vi "UV-VIS GetStatus.vi"(4 "error in (no error)":errorcluster, 7 "Detector in":refnum<class "CCD_camera.lvclass">) -> (0 "error out":errorcluster, 1 "DLL error code":u32, 2 "status":T1, 3 "Detector out":refnum<class "CCD_camera.lvclass">)   [LabVIEW 2018, in "CCD_camera.lvclass"]
doc: "This function will return the current status of the drivers. This function should be called before an acquisition is started to ensure that it is IDLE and during an acquisition to monitor the process.\n\n<B>Parameter:</B>\nstatus - current status\n DRV_IDLE - IDLE waiting on instructions.\n DRV_TEMPCYCLE - Executing temperature cycle.\n DRV_ACQUIRING - Acquisition in progress.\n DRV_ACCUM_TIME_NOT_MET - Unable to meet Accumulate cycle time.\n DRV_KINETIC_TIME_NOT_MET - Unable to meet Kinetic cycle time.\n DRV_ERROR_ACK - Unable to communicate with card.\n DRV_ACQ_BUFFER - Computer unable to read the data via the ISA slot at the required rate.\n\n<B>Error codes:</B>\nDRV_SUCCESS - Driver status return\nDRV_NOT_INITIALIZED - System not initialized\n\n<B>NOTES:</B>\n<B>If the status is DRV_ACCUM_TIME_NOT_MET, DRV_KINETIC_TIME_NOT_MET, DRV_ERROR_ACK or DRV_ACQ_BUFFER then the current acquisition will be aborted automatically.</B>"
uses:
  CCD_camera.lvclass
  dependecies/Error Code Enum typedef.ctl
  C:/Users/Sergey Denisov/Documents/REPS/TRANCON/Classes/Detector/Detector.lvclass
  Detector.lvclass/Detector.ctl
  Detector.lvclass
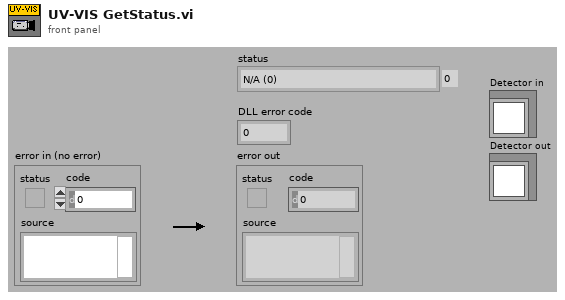
[diagram p1: front panel]
types:
  T1 = typedef "Error Code Enum typedef.ctl" = enum32{"N/A (0)", "DRV_ERROR_CODES", "DRV_SUCCESS", "DRV_VXDNOTINSTALLED", "DRV_ERROR_SCAN", "DRV_ERROR_CHECK_SUM", "DRV_ERROR_FILELOAD", "DRV_UNKNOWN_FUNC", "DRV_ERROR_VXD_INIT", "DRV_ERROR_ADDRESS", "DRV_ERROR_PAGELOCK", "DRV_ERROR_PAGEUNLOCK", "DRV_ERROR_BOARDTEST", "DRV_ERROR_ACK", "DRV_ERROR_UP_FIFO", "DRV_ERROR_PATTERN", "N/A (16)", "DRV_ACQUISITION_ERRORS", "DRV_ACQ_BUFFER", "DRV_ACQ_DOWNFIFO_FULL", "DRV_PROC_UNKONWN_INSTRUCTION", "DRV_ILLEGAL_OP_CODE", "DRV_KINETIC_TIME_NOT_MET", "DRV_ACCUM_TIME_NOT_MET", "DRV_NO_NEW_DATA", "N/A (25)", "DRV_SPOOLERROR", "N/A (27)", "N/A (28)", "N/A (29)", "N/A (30)", "N/A (31)", "N/A (32)", "DRV_TEMPERATURE_CODES", "DRV_TEMPERATURE_OFF", "DRV_TEMPERATURE_NOT_STABILIZED", "DRV_TEMPERATURE_STABILIZED", "DRV_TEMPERATURE_NOT_REACHED", "DRV_TEMPERATURE_OUT_RANGE", "DRV_TEMPERATURE_NOT_SUPPORTED", "DRV_TEMPERATURE_DRIFT", "N/A (41)", "N/A (42)", "N/A (43)", "N/A (44)", "N/A (45)", "N/A (46)", "N/A (47)", "N/A (48)", "DRV_GENERAL_ERRORS", "DRV_INVALID_AUX", "DRV_COF_NOTLOADED", "DRV_FPGAPROG", "DRV_FLEXERROR", "DRV_GPIBERROR", "N/A (55)", "N/A (56)", "N/A (57)", "N/A (58)", "N/A (59)", "N/A (60)", "N/A (61)", "N/A (62)", "N/A (63)", "DRV_DATATYPE", "DRV_DRIVER_ERRORS", "DRV_P1INVALID", "DRV_P2INVALID", "DRV_P3INVALID", "DRV_P4INVALID", "DRV_INIERROR", "DRV_COFERROR", "DRV_ACQUIRING", "DRV_IDLE", "DRV_TEMPCYCLE", "DRV_NOT_INITIALIZED", "DRV_P5INVALID", "DRV_P6INVALID", "DRV_INVALID_MODE", "DRV_INVALID_FILTER", "DRV_I2CERRORS", "DRV_I2CDEVNOTFOUND", "DRV_I2CTIMEOUT", "DRV_P7INVALID", "N/A (84)", "N/A (85)", "N/A (86)", "N/A (87)", "N/A (88)", "N/A (89)", "DRV_IOCERROR", "DRV_VRMVERSIONERROR"}
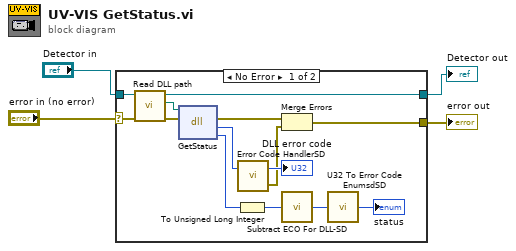
[diagram p0: block diagram]
diagram:
  n1 = case shown="No Error" "error in (no error)" {
    selector: "error in (no error)" -> [w12 w20]
    tunnel: [w8 w20] -> w3
    tunnel: [w5 w19] -> w2
    tunnel: "Detector in" -> [w6 w19]
    frame No Error {
      n2 = call "Read DLL path.vi"("error in (no error)"=w12, "Detector in"=w6) -> ("error out"=w11:errorcluster, "DLL path"=w7:path, "Detector out"=w5:refnum<class "CCD_camera.lvclass">)  [unwired: 7 in]
      n3 = dll-call lib="S:/TRANCON/DLL/Atmcd32d.dll" fn="GetStatus"(path in=w7, error in=w11) -> (error out=w10:errorcluster, "return type"=w18:u32, "status"=w16:i32)  [unwired: 2 in, 1 out]
      n4 = To Unsigned Long Integer(number=w16) -> (unsigned 32bit integer=w15:u32)
      n5 = call "Error Code HandlerSD.vi"("DLL error code"=w18) -> ("error out"=w9:errorcluster, "dup DLL error code"=→"DLL error code":u32)  [unwired: 1 in]
      n6 = Merge Errors(w10, w9) -> (w8:errorcluster)
      n7 = call "Subtract ECO For DLL-SD.vi"("x"=w15) -> ("x - ECO4DLL"=w14:u32)
      n8 = call "U32 To Error Code EnumsdSD.vi"("U32"=w14) -> ("error code enum"=→"status":T1)
    }
    frame Error {
    }
  }
  "error out" <- w3
  "Detector out" <- w2
